vi "TestData_OP-Comment.vi"(7 "Operation":enum16{"Add", "Remove", "Add-All", "Remove-All"}(ring), 8 "错误输入":errorcluster, 9 "Line Number":u32=1 min=1 step=1, 10 "Comment Mark":string, 11 "File Path":path) -> (0 "错误输出":errorcluster, 1 "Modified?":bool, 3 "ok?":bool)   [LabVIEW 2012, in "Lib_UEL.ATE.lvlib" / "Lib_TestData.lvlib"]
uses:
  Lib_TestData.lvlib
  <vilib>/Utility/file.llb/Read From Spreadsheet File (string).vi
  <vilib>/Utility/file.llb/Write To Spreadsheet File (string).vi
panel:
  # "功能说明:\n添加和删除注释到行首.\n添加注释: 自定义注释符合, 无论执行多少次, 只添加一个注释.\n删除注释: 自定义注释符合, 无论多少重复注释, 一次删除.\n\n版本信息: \nV1.0.0 初始版本. LiGuang@20151124"
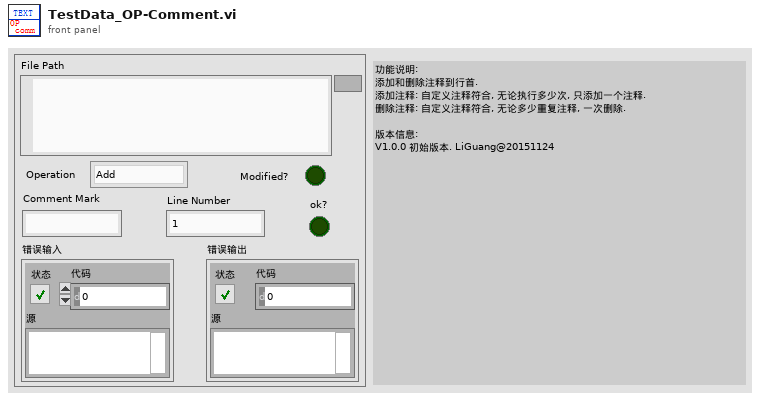
[diagram p1: front panel]
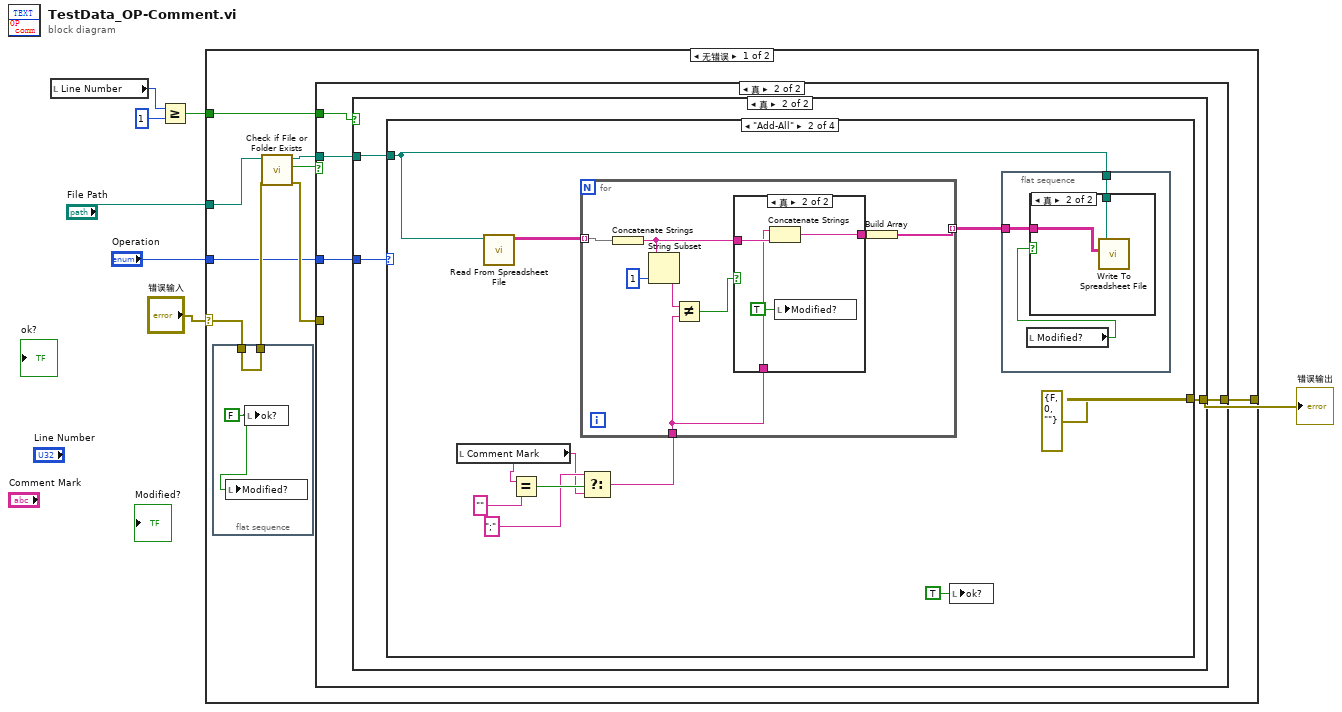
[diagram p0: block diagram]
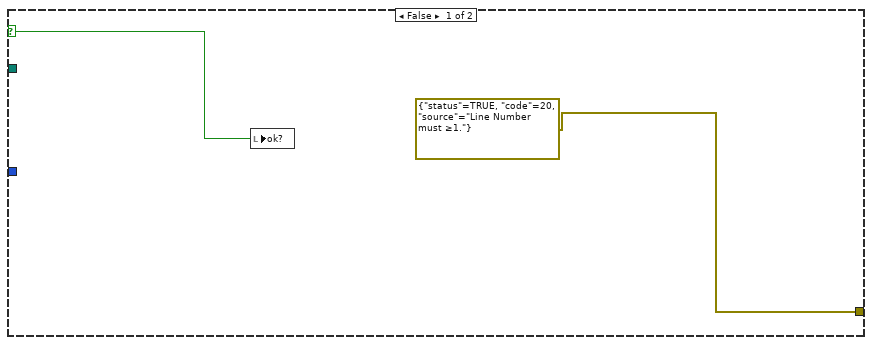
[diagram p3: hidden frame]
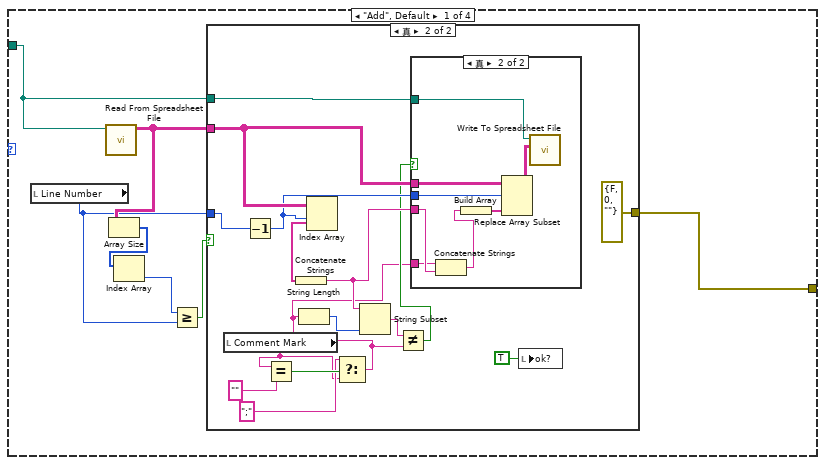
[diagram p4: hidden frame]
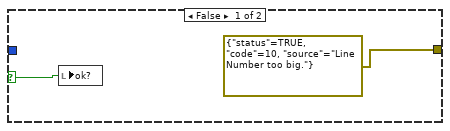
[diagram p5: hidden frame]
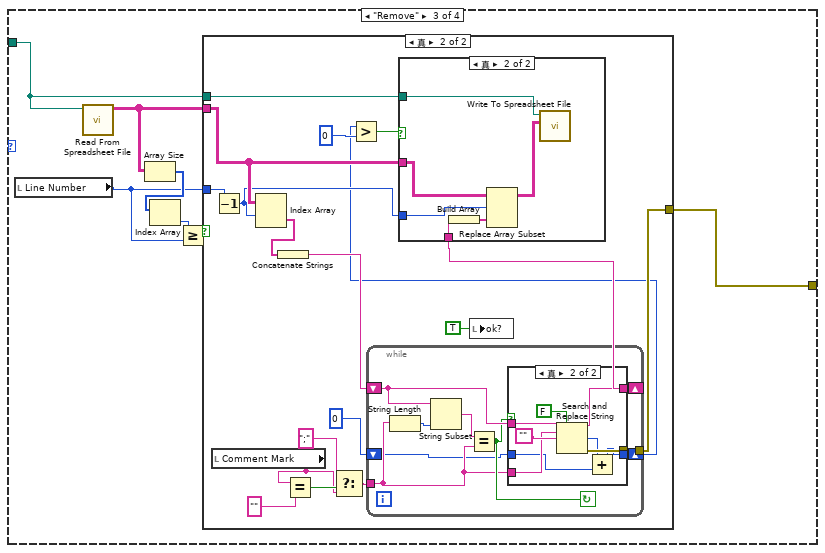
[diagram p9: hidden frame]
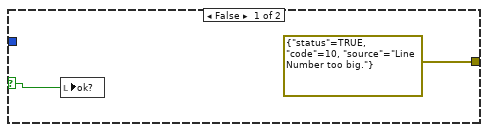
[diagram p10: hidden frame]
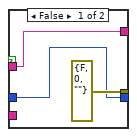
[diagram p11: hidden frame]
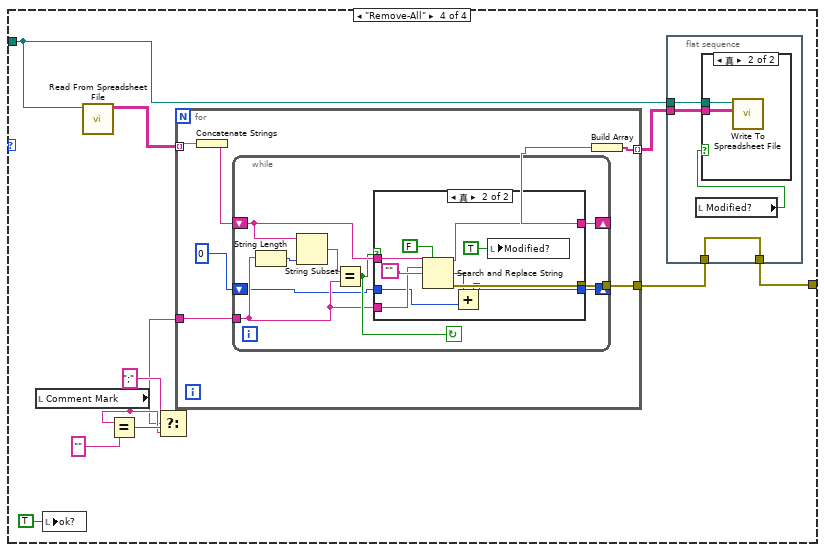
[diagram p13: hidden frame]
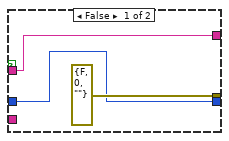
[diagram p15: hidden frame]
diagram:
  n1 = local read "Line Number"() -> (w3:u32)
  n2 = Greater Or Equal?(x=w3, y=u32 1) -> (x >= y?=w1:bool)
  n3 = case shown="无错误" "错误输入" {
    selector: "错误输入" -> [w10 w190]
    tunnel: "File Path" -> [w15 _]
    tunnel: [w16 w190] -> w6
    tunnel: "Operation" -> [w9 _]
    tunnel: w1 -> [w8 _]
    frame No Error {
      n4 = flat-sequence {
        tunnel: [w18] -> w11
        tunnel: w10 -> [w18]
        frame #0 {
          w17 = FALSE ("ok?")
          n5 = local write "Modified?"(w17) -> ()
          n6 = local write "ok?"(w17) -> ()
        }
      }
      n7 = call <vilib>:"Check if File or Folder Exists.vi"("error in (no error)"=w11, "path"=w15) -> ("error out"=w13:errorcluster, "file or folder exists?"=w14:bool, "dup path"=w12:path)  [unwired: 7 in]
      n8 = case shown="真" w14 {
        tunnel: w13 -> [w19 _]
        tunnel: [w19 w22] -> w16
        tunnel: w12 -> [_ w23]
        tunnel: w9 -> [_ w21]
        tunnel: w8 -> [_ w20]
        frame False {
        }
        frame True {
          n9 = case shown="真" w20 {
            selector: w20 -> [w25 _]
            tunnel: w23 -> [_ w28]
            tunnel: [errorcluster {"status"=TRUE, "code"=20, "source"="Line Number must ≥1."} ("error out") w27] -> w22
            tunnel: w21 -> [_ w26]
            frame False {
              n10 = local write "ok?"(w25) -> ()
            }
            frame True {
              n11 = case shown="\"Add-All\"" w26 {
                tunnel: w28 -> [w35 w62 w96 w154]
                tunnel: [w34 errorcluster {"status"=FALSE, "code"=0, "source"=""} ("error out") w95 w145] -> w27
                frame "Add", Default {
                  n12 = local read "Line Number"() -> (w29:u32)
                  n13 = call-poly <vilib>:"Read From Spreadsheet File.vi"("file path (dialog if empty)"=w35) -> ("all rows"=w32:string[][])  [unwired: 6 in, 4 out]
                  n14 = Array Size(array=w32) -> (size(s)=w33:i32[])
                  n15 = Index Array(array=w33) -> (element=w30:i32)  [unwired: 1 in]
                  n16 = Greater Or Equal?(x=w30, y=w29) -> (x >= y?=w31:bool)
                  n17 = case shown="真" w31 {
                    selector: w31 -> [w37 _]
                    tunnel: w35 -> [_ w52]
                    tunnel: [errorcluster {"status"=TRUE, "code"=10, "source"="Line Number too big."} ("error out") errorcluster {"status"=FALSE, "code"=0, "source"=""} ("error out")] -> w34
                    tunnel: w32 -> [_ w48]
                    tunnel: w29 -> [_ w47]
                    frame False {
                      n18 = local write "ok?"(w37) -> ()
                    }
                    frame True {
                      n19 = local read "Comment Mark"() -> (w38:string)
                      n20 = Decrement(x=w47) -> (x-1=w46:u32)
                      n21 = Equal?(x=w38, y="") -> (x = y?=w50:bool)
                      n22 = Index Array(array=w48, index (row)=w46) -> (element=w53:string[])  [unwired: 1 in]
                      n23 = Concatenate Strings(w53) -> (w45:string)
                      n24 = Select(t=";", s=w50, f=w38) -> (s? t:f=w39:string)
                      n25 = String Length(string=w39) -> (length=w44:i32)
                      n26 = String Subset(string=w45, length (rest)=w44) -> (substring=w43:string)  [unwired: 1 in]
                      n27 = Not Equal?(x=w43, y=w39) -> (x != y?=w42:bool)
                      n28 = case shown="真" w42 {
                        tunnel: w52 -> [_ w60]
                        tunnel: w48 -> [_ w58]
                        tunnel: w46 -> [_ w57]
                        tunnel: w45 -> [_ w56]
                        tunnel: w39 -> [_ w55]
                        frame False {
                        }
                        frame True {
                          n29 = Concatenate Strings(w55, w56) -> (w54:string)
                          n30 = Build Array(w54) -> (w61:string[])
                          n31 = Replace Array Subset(array=w58, new element=w61, index (row)=w57) -> (w59:string[][])  [unwired: 1 in]
                          n32 = call-poly <vilib>:"Write To Spreadsheet File.vi"("2D data"=w59, "file path (dialog if empty)"=w60) -> ()  [unwired: 6 in, 1 out]
                        }
                      }
                      n33 = local write "ok?"(TRUE ("ok?")) -> ()
                    }
                  }
                }
                frame "Add-All" {
                  n34 = local read "Comment Mark"() -> (w66:string)
                  n35 = call-poly <vilib>:"Read From Spreadsheet File.vi"("file path (dialog if empty)"=w62) -> ("all rows"=w65:string[][])  [unwired: 6 in, 4 out]
                  n36 = Equal?(x=w66, y="") -> (x = y?=w69:bool)
                  n37 = Select(t=";", s=w69, f=w66) -> (s? t:f=w64:string)
                  n38 = for {
                    tunnel: w65 -> [w84] mode=indexing
                    tunnel: w64 -> [w78]
                    tunnel: [w82] -> w63 mode=indexing
                    n39 = Concatenate Strings(w84) -> (w81:string)
                    n40 = String Subset(string=w81, length (rest)=1 ("长度（剩余）")) -> (substring=w79:string)  [unwired: 1 in]
                    n41 = Not Equal?(x=w79, y=w78) -> (x != y?=w77:bool)
                    n42 = case shown="真" w77 {
                      tunnel: [w85 w89] -> w83
                      tunnel: w81 -> [w85 w88]
                      tunnel: w78 -> [_ w87]
                      frame False {
                      }
                      frame True {
                        n43 = Concatenate Strings(w87, w88) -> (w89:string)
                        n44 = local write "Modified?"(TRUE ("Modified?")) -> ()
                      }
                    }
                    n45 = Build Array(w83) -> (w82:string[])
                  }
                  n46 = local write "ok?"(TRUE ("ok?")) -> ()
                  n47 = flat-sequence {
                    tunnel: w63 -> [w74]
                    tunnel: w62 -> [w73]
                    frame #0 {
                      n48 = local read "Modified?"() -> (w72:bool)
                      n49 = case shown="真" w72 {
                        tunnel: w74 -> [_ w76]
                        tunnel: w73 -> [_ w75]
                        frame False {
                        }
                        frame True {
                          n50 = call-poly <vilib>:"Write To Spreadsheet File.vi"("2D data"=w76, "file path (dialog if empty)"=w75) -> ()  [unwired: 6 in, 1 out]
                        }
                      }
                    }
                  }
                }
                frame "Remove" {
                  n51 = local read "Line Number"() -> (w90:u32)
                  n52 = call-poly <vilib>:"Read From Spreadsheet File.vi"("file path (dialog if empty)"=w96) -> ("all rows"=w94:string[][])  [unwired: 6 in, 4 out]
                  n53 = Array Size(array=w94) -> (size(s)=w93:i32[])
                  n54 = Index Array(array=w93) -> (element=w91:i32)  [unwired: 1 in]
                  n55 = Greater Or Equal?(x=w91, y=w90) -> (x >= y?=w92:bool)
                  n56 = case shown="真" w92 {
                    selector: w92 -> [w98 _]
                    tunnel: w96 -> [_ w115]
                    tunnel: [errorcluster {"status"=TRUE, "code"=10, "source"="Line Number too big."} ("error out") w110] -> w95
                    tunnel: w94 -> [_ w107]
                    tunnel: w90 -> [_ w106]
                    frame False {
                      n57 = local write "ok?"(w98) -> ()
                    }
                    frame True {
                      n58 = local read "Comment Mark"() -> (w111:string)
                      n59 = Decrement(x=w106) -> (x-1=w105:u32)
                      n60 = Index Array(array=w107, index (row)=w105) -> (element=w116:string[])  [unwired: 1 in]
                      n61 = Concatenate Strings(w116) -> (w103:string)
                      n62 = Equal?(x=w111, y="") -> (x = y?=w113:bool)
                      n63 = Select(t=";", s=w113, f=w111) -> (s? t:f=w104:string)
                      n64 = while {
                        tunnel: [w125] -> w110
                        tunnel: w104 -> [w119]
                        shift-right: [w121] -> w102
                        shift-left: w103 -> [w122]
                        shift-right: [w117] -> w100
                        shift-left: 0 -> [w118]
                        stop <- w120 continue-if-true
                        n65 = String Length(string=w119) -> (length=w124:i32)
                        n66 = String Subset(string=w122, length (rest)=w124) -> (substring=w123:string)  [unwired: 1 in]
                        n67 = Equal?(x=w123, y=w119) -> (x = y?=w120:bool)
                        n68 = case shown="真" w120 {
                          tunnel: [errorcluster {"status"=FALSE, "code"=0, "source"=""} ("error out") w135] -> w125
                          tunnel: w122 -> [w128 w134]
                          tunnel: [w128 w133] -> w121
                          tunnel: w119 -> [_ w132]
                          tunnel: w118 -> [w126 w130]
                          tunnel: [w126 w129] -> w117
                          frame False {
                          }
                          frame True {
                            n69 = Search and Replace String(replace all?=FALSE ("替换全部？(F)"), input string=w134, search string=w132, replace string="") -> (result string=w133:string, number of replacements=w131:i32, error out=w135:errorcluster)  [unwired: 4 in, 1 out]
                            n70 = Add(x=w131, y=w130) -> (x+y=w129:i32)
                          }
                        }
                      }
                      n71 = Greater?(x=w100, y=0) -> (0:w108:bool)
                      n72 = case shown="真" w108 {
                        tunnel: w107 -> [_ w143]
                        tunnel: w115 -> [_ w142]
                        tunnel: w105 -> [_ w140]
                        tunnel: w102 -> [_ w139]
                        frame False {
                        }
                        frame True {
                          n73 = Build Array(w139) -> (w138:string[])
                          n74 = Replace Array Subset(array=w143, new element=w138, index (row)=w140) -> (w141:string[][])  [unwired: 1 in]
                          n75 = call-poly <vilib>:"Write To Spreadsheet File.vi"("2D data"=w141, "file path (dialog if empty)"=w142) -> ()  [unwired: 6 in, 1 out]
                        }
                      }
                      n76 = local write "ok?"(TRUE ("ok?")) -> ()
                    }
                  }
                }
                frame "Remove-All" {
                  n77 = local read "Comment Mark"() -> (w150:string)
                  n78 = local write "ok?"(TRUE ("ok?")) -> ()
                  n79 = call-poly <vilib>:"Read From Spreadsheet File.vi"("file path (dialog if empty)"=w154) -> ("all rows"=w147:string[][])  [unwired: 6 in, 4 out]
                  n80 = Equal?(x=w150, y="") -> (x = y?=w152:bool)
                  n81 = Select(t=";", s=w152, f=w150) -> (s? t:f=w149:string)
                  n82 = for {
                    tunnel: [w167] -> w144
                    tunnel: w149 -> [w166]
                    tunnel: w147 -> [w164] mode=indexing
                    tunnel: [w161] -> w146 mode=indexing
                    n83 = Concatenate Strings(w164) -> (w163:string)
                    n84 = while {
                      tunnel: [w176] -> w167
                      tunnel: w166 -> [w170]
                      shift-right: [w172] -> w162
                      shift-left: w163 -> [w173]
                      shift-right: [w168] -> _
                      shift-left: 0 -> [w169]
                      stop <- w171 continue-if-true
                      n85 = String Length(string=w170) -> (length=w175:i32)
                      n86 = String Subset(string=w173, length (rest)=w175) -> (substring=w174:string)  [unwired: 1 in]
                      n87 = Equal?(x=w174, y=w170) -> (x = y?=w171:bool)
                      n88 = case shown="真" w171 {
                        tunnel: [errorcluster {"status"=FALSE, "code"=0, "source"=""} ("error out") w187] -> w176
                        tunnel: w173 -> [w179 w186]
                        tunnel: [w179 w185] -> w172
                        tunnel: w170 -> [_ w184]
                        tunnel: w169 -> [w177 w182]
                        tunnel: [w177 w181] -> w168
                        frame False {
                        }
                        frame True {
                          n89 = Search and Replace String(replace all?=FALSE ("替换全部？(F)"), input string=w186, search string=w184, replace string="") -> (result string=w185:string, number of replacements=w183:i32, error out=w187:errorcluster)  [unwired: 4 in, 1 out]
                          n90 = Add(x=w183, y=w182) -> (x+y=w181:i32)
                          n91 = local write "Modified?"(TRUE ("Modified?")) -> ()
                        }
                      }
                    }
                    n92 = Build Array(w162) -> (w161:string[])
                  }
                  n93 = flat-sequence {
                    tunnel: w154 -> [w158]
                    tunnel: w146 -> [w157]
                    tunnel: [w156] -> w145
                    tunnel: w144 -> [w156]
                    frame #0 {
                      n94 = local read "Modified?"() -> (w155:bool)
                      n95 = case shown="真" w155 {
                        tunnel: w158 -> [_ w160]
                        tunnel: w157 -> [_ w159]
                        frame False {
                        }
                        frame True {
                          n96 = call-poly <vilib>:"Write To Spreadsheet File.vi"("2D data"=w159, "file path (dialog if empty)"=w160) -> ()  [unwired: 6 in, 1 out]
                        }
                      }
                    }
                  }
                }
              }
            }
          }
        }
      }
    }
    frame Error {
    }
  }
  "错误输出" <- w6
